vi "SLSC Queue Command.vi"(8 "error in":errorcluster, 9 "CS Bits":T4={"CS Bit 1"="Connector0/DIO0", "CS Bit 2"="Connector0/DIO0", "CS Bit 3"="Connector0/DIO0", "CS Bit 4"="Connector0/DIO0"}, 10 "SLSC SPI Command":T1={"Chip Select"=0, "CS Bit Value/Slot #"=0, "SPI PHY Settings"={"Divide Value"=0, "Transfer Length (bits)"=1, "CS Asserted Polarity"=FALSE, "Clock Polarity (CPOL)"=FALSE, "Clock Phase (CPHA)"=FALSE, "Lengthen MISO Setup"=FALSE, "Direction Change Bit"=0, "MOSI Starts as Output"=FALSE, "Tristatable MOSI"=FALSE}, "Data to DAC"=0} {"SPI PHY Settings"."Direction Change Bit" max=64 step=1; "SPI PHY Settings"."Transfer Length (bits)" min=1 max=64 step=1}, 11 "SPI API References":T3={"DLU To SPI Engine Data FIFO"="DLU To SPI Engine Data", "SPI Engine to DLU Data FIFO"="SPI Engine to DLU Data", "Data to SPI Engine (Cache) Register"="Data to SPI Engine (Cache)", "SPI PHY Settings to SPI Engine (Cahche) Register"="SPI PHY Settings to SPI Engine (Cache)"}) -> (0 "error out":errorcluster, 2 "read Iterations":i32, 3 "Data to Node":u64)   [LabVIEW 2014, in "SLSC FPGA Toolkit.lvlib"]
uses:
  SLSC FPGA Toolkit.lvlib
  <vilib>/Platform/TimedLoop/XDataNode/wakeup.ctl
  <vilib>/Platform/TimedLoop/XDataNode/XDNodeRunTimeDep.lvlib
  <vilib>/Platform/TimedLoop/XDataNode/nitl_modes.ctl
  <vilib>/Platform/TimedLoop/XDataNode/timing_clust.ctl
  <vilib>/Platform/TimedLoop/XDataNode/XDataNode.xnode
  CD/Source/Shared/SPI Utility/CS Bits.ctl
  CD/Source/Shared/SLSC configuration Shared.lvlib
  <userlib>/_NI SPI IP/FPGA/Controllers/Public/Transfer Settings.ctl
  <userlib>/_NI SPI IP/FPGA/Controllers/NI SPI IP FPGA.lvlib
  <vilib>/SPI API/SPIAPI/Controls/Internal Data (SPI API).ctl
  SLSC SPI Command.ctl
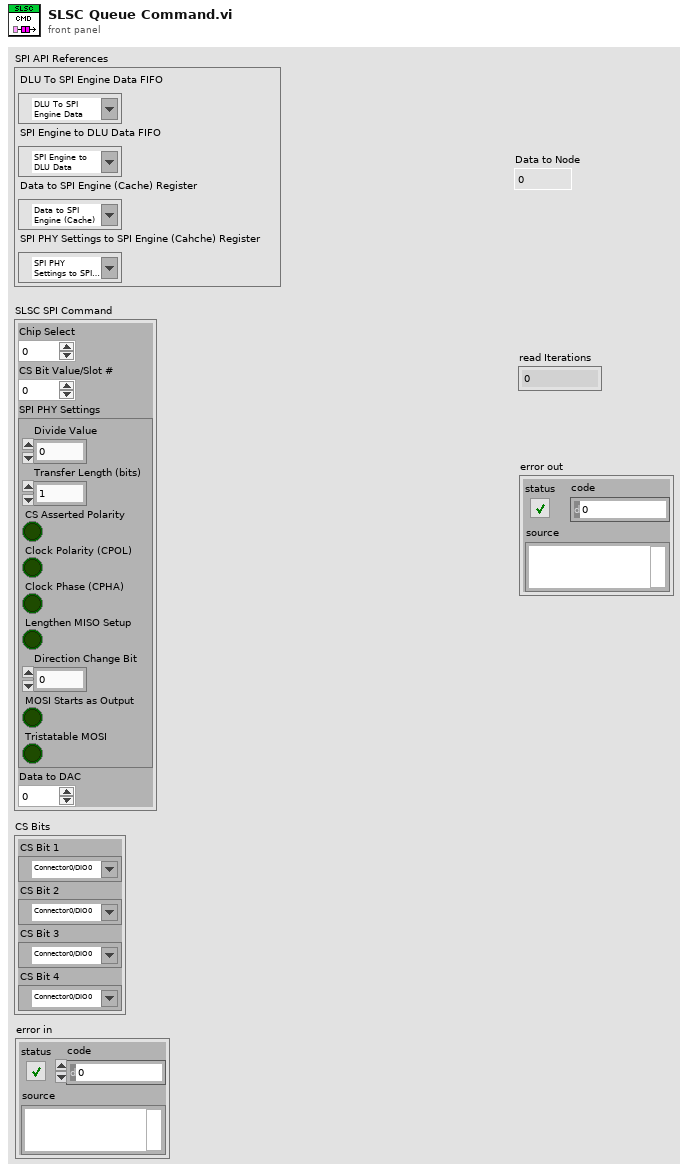
[diagram p1: front panel]
types:
  T1 = typedef "SLSC FPGA Toolkit.lvlib/SLSC SPI Command.ctl" = cluster{"Chip Select":u8, "CS Bit Value/Slot #":u8, "SPI PHY Settings":T2, "Data to DAC":u64}
  T2 = typedef "NI SPI IP FPGA.lvlib/Transfer Settings.ctl" = cluster{"Divide Value":u8, "Transfer Length (bits)":u8, "CS Asserted Polarity":bool, "Clock Polarity (CPOL)":bool, "Clock Phase (CPHA)":bool, "Lengthen MISO Setup":bool, "Direction Change Bit":u8, "MOSI Starts as Output":bool, "Tristatable MOSI":bool}
  T3 = typedef "Internal Data (SPI API).ctl" = cluster{"DLU To SPI Engine Data FIFO":refnum<k21>, "SPI Engine to DLU Data FIFO":refnum<k21>, "Data to SPI Engine (Cache) Register":refnum<k21>, "SPI PHY Settings to SPI Engine (Cahche) Register":refnum<k21>}
  T4 = typedef "SLSC configuration Shared.lvlib/CS Bits.ctl" = cluster{"CS Bit 1":refnum<k21>, "CS Bit 2":refnum<k21>, "CS Bit 3":refnum<k21>, "CS Bit 4":refnum<k21>}
  T5 = typedef "XDNodeRunTimeDep.lvlib/timing_clust.ctl" = cluster{"Expected End [f-1]":u64, "Actual End [f-1]":u64, "Finished Late? [f-1]":bool, "Expected End [i-1]":u64, "Actual End [i-1]":u64, "Finished Late? [i-1]":bool, "Expected Start [i]":u64, "Actual Start [i]":u64, "Expected Start [f]":u64, "Actual Start [f]":u64, "Source Name":string, "Structure Name":string, "Period":i64, "Deadline":i64, "Offset":i64, "Start":i64, "Priority":i32, "Timeout":i32, "Mode":T6, "Wakeup Reason":T7, "Error":errorcluster, "Source Type":string, "Secondary Source Type":string, "Global End Time":u64, "Global Start Time":u64, "Frame Duration":u64, "Iteration Duration":u64, "Assigned CPU":i32, "I/O Scan Engine Mode":u32}
  T6 = typedef "XDNodeRunTimeDep.lvlib/nitl_modes.ctl" = enum32{"No Change", "Process missed periods, maintain original phase", "Discard missed periods, maintain original phase", "Process missed periods, ignore original phase", "Discard missed periods, ignore original phase"}
  T7 = typedef "XDNodeRunTimeDep.lvlib/wakeup.ctl" = enum32{"Normal", "Aborted", "Asynchronous wakeup", "Timing source error", "Timed loop error", "Timeout"}
  T8 = typedef "SPI Response Information.ctl" = cluster{"Data to Node":u64, "Node Id":u16}
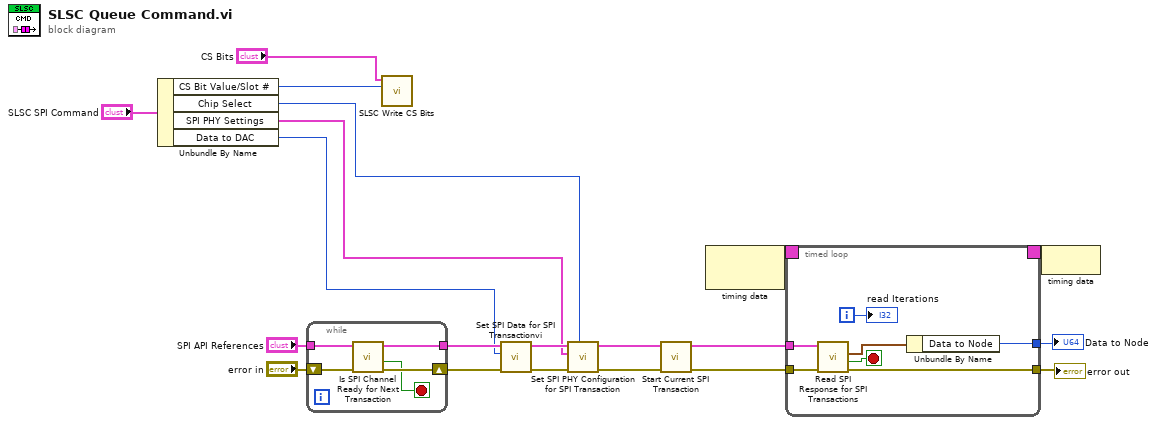
[diagram p0: block diagram]
diagram:
  n1 = Unbundle By Name("SLSC SPI Command") -> ("CS Bit Value/Slot #"=w2:u8, "Chip Select"=w5:u8, "SPI PHY Settings"=w4:T2, "Data to DAC"=w3:u64)
  n2 = while {
    shift-right: [w25] -> w18
    shift-left: "error in" -> [w23]
    tunnel: "SPI API References" -> [w21]
    tunnel: [w24] -> w17
    stop <- w22 stop-if-true
    n3 = call <vilib>:"Is SPI Channel Ready for Next Transaction.vi"("error in"=w23, "Private Data In"=w21) -> ("error out"=w25:errorcluster, "SPI Channel Ready"=w22:bool, "Private Data Out"=w24:T3)  [unwired: 6 in, 1 out]
  }
  n4 = call "SLSC Write CS Bits.vi"("CS Bit Value/Slot #"=w2, "CS Bits"="CS Bits") -> ()  [unwired: 10 in]
  n5 = call <vilib>:"Set SPI Data for SPI Transactionvi.vi"("error in"=w18, "Data In"=w3, "Private Data In"=w17) -> ("error out"=w14:errorcluster, "Private Data Out"=w15:T3)  [unwired: 7 in]
  n6 = call <vilib>:"Set SPI PHY Configuration for SPI Transaction.vi"("Chip Select"=w5, "error in"=w14, "SPI PHY Settings"=w4, "Private Data In"=w15) -> ("error out"=w12:errorcluster, "Private Data Out"=w13:T3)  [unwired: 6 in]
  n7 = call <vilib>:"Start Current SPI Transaction.vi"("error in"=w12, "Private Data In"=w13) -> ("error out"=w16:errorcluster, "Private Data Out"=w11:T3)  [unwired: 7 in, 1 out]
  n8 = node-c288() -> (w20:T5)  [unwired: 1 in]
  n9 = timed-loop {
    timing: w20 -> [_]
    timing-out: [_] -> w19
    tunnel: w16 -> [w32]
    tunnel: w11 -> [w31]
    tunnel: [w26] -> w9
    tunnel: [w28] -> w8
    i -> [w27]
    stop <- w30 stop-if-true
    n10 = call <vilib>:"Read SPI Response for SPI Transactions.vi"("error in"=w32, "Private Data In"=w31) -> ("error out"=w28:errorcluster, "Read Data Valid?"=w30:bool, "Read Data"=w29:T8)  [unwired: 6 in, 1 out]
    n11 = Unbundle By Name(w29) -> ("Data to Node"=w26:u64)
    "read Iterations" <- w27
  }
  "Data to Node" <- w9
  "error out" <- w8
  n12 = node-c288(w19) -> ()
